vi "LabVIEW Gaussian Signal Monitor with UDP Alert System.vi"() -> ()   [LabVIEW 2024]
uses:
  Pro. Cases.ctl
  Con. Cases.ctl
  <vilib>/Utility/file.llb/Write Delimited Spreadsheet (DBL).vi
panel:
  out "error out":errorcluster
  in  "S. Freq. (Hz)":dbl=10.0 min=10.0 max=200.0
  out "Triggered Data":dbl[](graph)
  out "Real Time":dbl(graph)
  in  "L (V)":dbl=0.0001 min=0.0001 max=0.9999
  in  "W (s)":dbl min=1.0001
  in  "K (s)":dbl min=0.0001
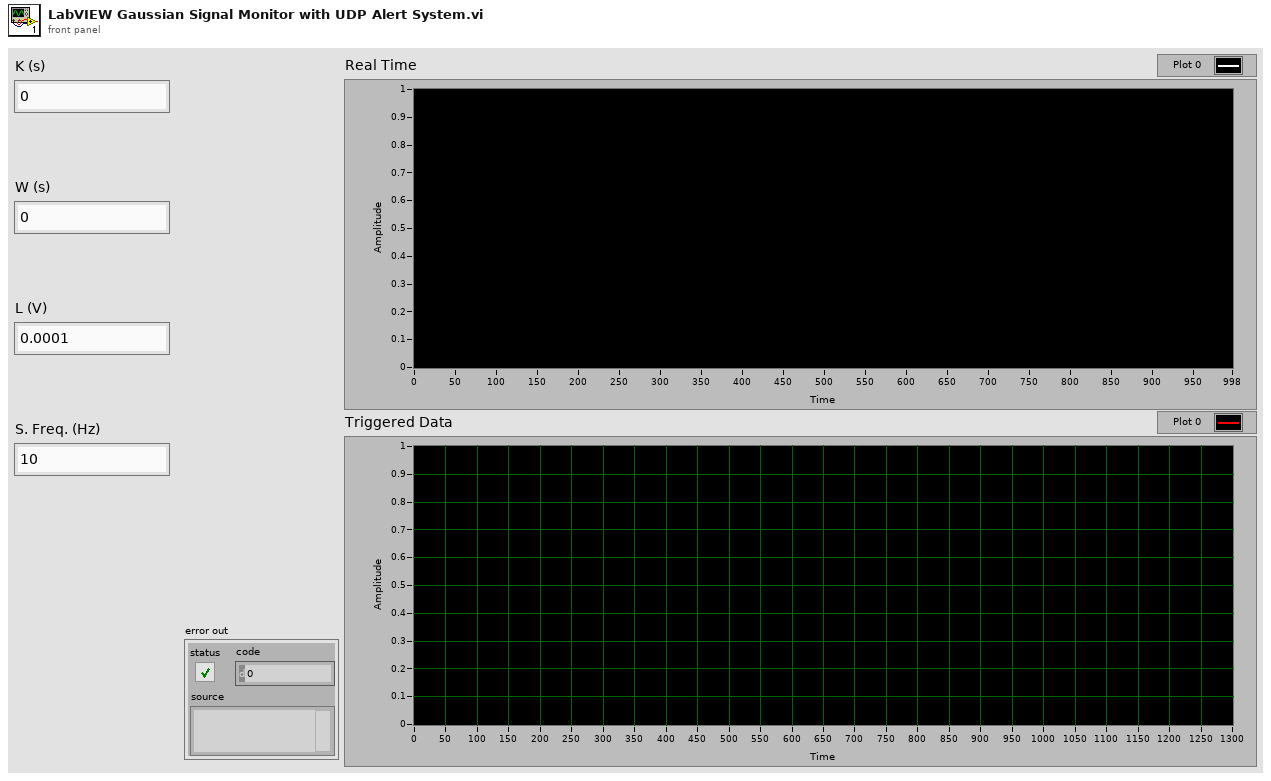
[diagram p1: front panel]
types:
  T1 = typedef "Con. Cases.ctl" = enum16{"Transmission", "Stop"}
  T2 = enum16{"open", "replace", "create", "open or create", "replace or create", "replace or create with confirmation"}
  T3 = typedef "Pro. Cases.ctl" = enum16{"Poll", "Acq.", "Save", "Stop"}
  T4 = cluster{"Pro. Cases":T3, "W (s)":dbl, "L (V)":dbl, "K (s)":dbl, "S. Freq. (Hz)":dbl, "i":dbl, "x (t)":dbl, "Trg.":bool, "counter":i32, "Trg. F.":dbl[], "File":refnum<file>}
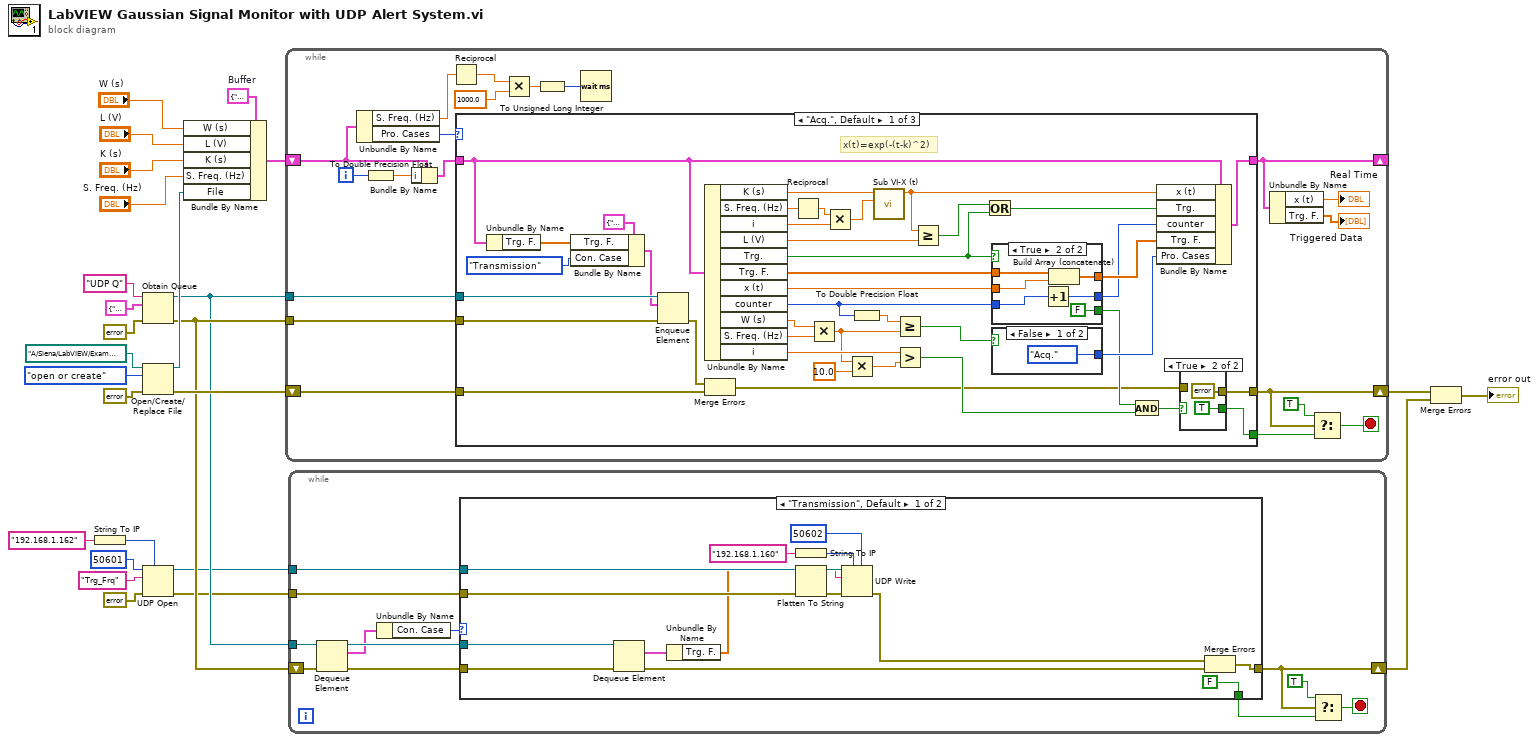
[diagram p0: block diagram]
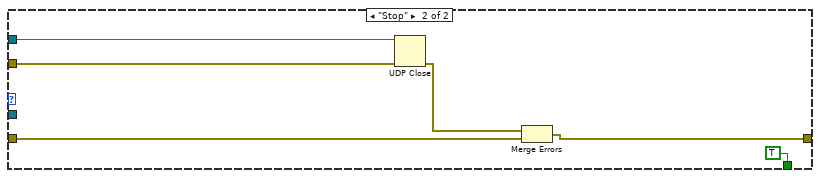
[diagram p2: hidden frame]
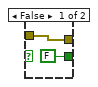
[diagram p3: hidden frame]
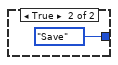
[diagram p4: hidden frame]
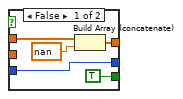
[diagram p5: hidden frame]
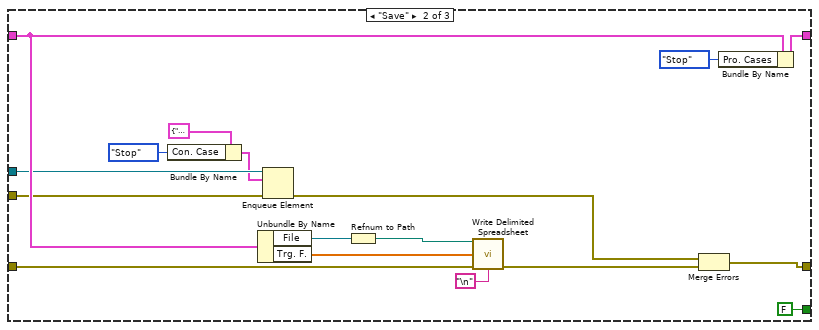
[diagram p6: hidden frame]
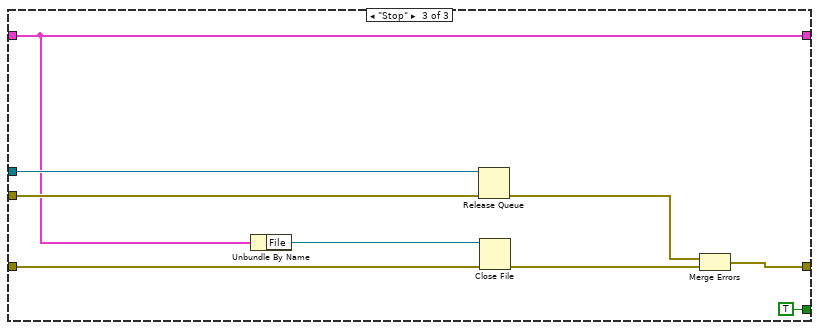
[diagram p7: hidden frame]
diagram:
  w26 = T4 {"Pro. Cases"=enum."Acq.", "W (s)"=0.0, "L (V)"=0.0, "K (s)"=0.0, "S. Freq. (Hz)"=0.0, "i"=0.0, "x (t)"=0.0, "Trg."=FALSE, "counter"=0, "Trg. F."=[], "File"=refnum}  # Buffer
  n1 = String To IP(1:"192.168.1.162" ("name")) -> (0:w2:u32)
  n2 = Obtain Queue(name (unnamed)="UDP Q", element data type=cluster{"Con. Case":T1, "Trg. F.":dbl[]} {"Con. Case"=enum."Transmission", "Trg. F."=[]}, error in (no error)=errorcluster {"status"=FALSE, "code"=0, "source"=""} ("error in")) -> (queue out=w11:refnum<queue>, error out=w12:errorcluster)  [unwired: 2 in, 1 out]
  n3 = Open/Create/Replace File(file path (use dialog)=path "A:/Siena/LabVIEW/Exam Perp/Triggered Data/Trg data.csv", error in=errorcluster {"status"=FALSE, "code"=0, "source"=""}, operation (0:open)=T2."open or create") -> (refnum out=w16:refnum<file>, error out=w17:errorcluster)  [unwired: 3 in, 1 out]
  n4 = UDP Open(7:w2, 8:errorcluster {"status"=FALSE, "code"=0, "source"=""} ("error in"), 10:"Trg_Frq" ("service name"), 11:u16 50601 ("port")) -> (port=w7:refnum<k16>, 0:w6:errorcluster)  [unwired: 1 in, 1 out]
  n5 = Bundle By Name(cluster=w26, "W (s)"="W (s)", "L (V)"="L (V)", "K (s)"="K (s)", "S. Freq. (Hz)"="S. Freq. (Hz)", "File"=w16) -> (w25:T4)
  n6 = while {
    shift-right: [w36] -> _
    shift-left: w25 -> [w40]
    shift-right: [w32] -> w15
    shift-left: w17 -> [w33]
    tunnel: w11 -> [w28]
    tunnel: w12 -> [w27]
    i -> [w46]
    stop <- w29 stop-if-true
    n7 = Unbundle By Name(w40) -> ("S. Freq. (Hz)"=w41:dbl, "Pro. Cases"=w38:T3)
    n8 = To Double Precision Float(number=w46) -> (double precision float=w37:dbl)
    n9 = Bundle By Name(cluster=w40, "i"=w37) -> (w39:T4)
    n10 = Reciprocal(x=w41) -> (1/x=w42:dbl)
    n11 = case shown="\"Acq.\", Default" w38 {
      tunnel: w39 -> [w49 w120 w121]
      tunnel: [w80 w119 w121] -> w36
      tunnel: w33 -> [w54 w116 w129]
      tunnel: [w63 w104 w122] -> w32
      tunnel: [w62 FALSE TRUE] -> w30
      tunnel: w28 -> [w56 w111 w126]
      tunnel: w27 -> [w55 w110 w125]
      frame "Acq.", Default {
        # "x(t)=exp(-(t-k)^2)"
        n12 = Unbundle By Name(w49) -> ("Trg. F."=w48:dbl[])
        n13 = Bundle By Name(cluster=cluster{"Con. Case":T1, "Trg. F.":dbl[]} {"Con. Case"=enum."Transmission", "Trg. F."=[]}, "Trg. F."=w48, "Con. Case"=Con._Cases."Transmission") -> (w50:cluster{"Con. Case":T1, "Trg. F.":dbl[]})
        n14 = Enqueue Element(queue=w56, element=w50, error in (no error)=w55) -> (error out=w52:errorcluster)  [unwired: 1 in, 2 out]
        n15 = Unbundle By Name(w49) -> ("K (s)"=w85:dbl, "S. Freq. (Hz)"=w84:dbl, "i"=w81:dbl, "L (V)"=w79:dbl, "Trg."=w76:bool, "Trg. F."=w73:dbl[], "x (t)"=w72:dbl, "counter"=w69:i32, "W (s)"=w71:dbl, "S. Freq. (Hz)"=w70:dbl, "i"=w61:dbl)
        n16 = Merge Errors(w52, w54) -> (w53:errorcluster)
        n17 = Reciprocal(x=w84) -> (1/x=w83:dbl)
        n18 = Multiply(x=w71, y=w70) -> (x*y=w57:dbl)
        n19 = Multiply(x=w83, y=w81) -> (x*y=w82:dbl)
        n20 = Multiply(x=w57, y=10.0) -> (x*y=w64:dbl)
        n21 = To Double Precision Float(number=w69) -> (double precision float=w65:dbl)
        n22 = call "Sub VI-X (t).vi"("t"=w82, "K"=w85) -> ("x (t)"=w74:dbl)  [unwired: 8 in, 1 out]
        n23 = Greater Or Equal?(x=w65, y=w57) -> (x >= y?=w68:bool)
        n24 = Greater?(x=w61, y=w64) -> (0:w58:bool)
        n25 = Greater Or Equal?(x=w74, y=w79) -> (x >= y?=w78:bool)
        n26 = Or(x=w78, y=w76) -> (x .or. y?=w77:bool)
        n27 = case shown="True" w76 {
          tunnel: w69 -> [w97 w103]
          tunnel: [w97 w102] -> w75
          tunnel: w73 -> [w95 w101]
          tunnel: [w96 w100] -> w86
          tunnel: w72 -> [_ w99]
          tunnel: [TRUE FALSE] -> w59
          frame False {
            n28 = Build Array (concatenate)(w95, nan) -> (w96:dbl[])
          }
          frame True {
            n29 = Increment(x=w103) -> (x+1=w102:i32)
            n30 = Build Array (concatenate)(w101, w99) -> (w100:dbl[])
          }
        }
        n31 = case shown="False" w68 {
          tunnel: [Pro._Cases."Acq." ("Cases") Pro._Cases."Save" ("Cases")] -> w67
          frame False {
          }
          frame True {
          }
        }
        n32 = And(x=w59, y=w58) -> (x .and. y?=w60:bool)
        n33 = Bundle By Name(cluster=w49, "x (t)"=w74, "Trg."=w77, "counter"=w75, "Trg. F."=w86, "Pro. Cases"=w67) -> (w80:T4)
        n34 = case shown="True" w60 {
          tunnel: w53 -> [w88 _]
          tunnel: [w88 errorcluster {"status"=TRUE, "code"=5050, "source"="Waiting for trigger timeout error"} ("error out")] -> w63
          tunnel: [FALSE TRUE] -> w62
          frame False {
          }
          frame True {
          }
        }
      }
      frame "Save" {
        n35 = Bundle By Name(cluster=cluster{"Con. Case":T1, "Trg. F.":dbl[]} {"Con. Case"=enum."Transmission", "Trg. F."=[]} ("element"), "Con. Case"=Con._Cases."Stop") -> (w108:cluster{"Con. Case":T1, "Trg. F.":dbl[]})
        n36 = Unbundle By Name(w120) -> ("File"=w115:refnum<file>, "Trg. F."=w113:dbl[])
        n37 = Enqueue Element(queue=w111, element=w108, error in (no error)=w110) -> (error out=w105:errorcluster)  [unwired: 1 in, 2 out]
        n38 = Refnum to Path(1:w115) -> (0:w114:path)
        n39 = call-poly <vilib>:"Write Delimited Spreadsheet.vi"("file path (dialog if empty)"=w114, "1D data"=w113, "error in (no error)"=w116, "delimiter (\\t)"="\n") -> ("error out"=w106:errorcluster)  [unwired: 10 in, 1 out]
        n40 = Merge Errors(w105, w106) -> (w104:errorcluster)
        n41 = Bundle By Name(cluster=w120, "Pro. Cases"=Pro._Cases."Stop" ("Cases")) -> (w119:T4)
      }
      frame "Stop" {
        n42 = Unbundle By Name(w121) -> ("File"=w128:refnum<file>)
        n43 = Release Queue(queue=w126, error in (no error)=w125) -> (error out=w124:errorcluster)  [unwired: 1 in, 2 out]
        n44 = Close File(refnum=w128, error in=w129) -> (error out=w123:errorcluster)  [unwired: 1 out]
        n45 = Merge Errors(w124, w123) -> (w122:errorcluster)
      }
    }
    n46 = Multiply(x=w42, y=1000.0) -> (x*y=w45:dbl)
    n47 = To Unsigned Long Integer(number=w45) -> (unsigned 32bit integer=w44:u32)
    n48 = Wait (ms)(milliseconds to wait=w44) -> ()  [unwired: 1 out]
    n49 = Unbundle By Name(w36) -> ("x (t)"=→"Real Time":dbl, "Trg. F."=→"Triggered Data":dbl[])
    n50 = Select(t=TRUE, s=w32, f=w30) -> (s? t:f=w29:bool)
  }
  n51 = while {
    tunnel: w11 -> [w140]
    tunnel: w7 -> [w131]
    tunnel: w6 -> [w130]
    shift-right: [w135] -> w8
    shift-left: w12 -> [w141]
    stop <- w134 stop-if-true
    n52 = Dequeue Element(queue=w140, error in (no error)=w141) -> (queue out=w139:refnum<queue>, element=w137:cluster{"Con. Case":T1, "Trg. F.":dbl[]}, error out=w138:errorcluster)  [unwired: 1 in, 1 out]
    n53 = Unbundle By Name(w137) -> ("Con. Case"=w136:T1)
    n54 = case shown="\"Transmission\", Default" w136 {
      tunnel: w139 -> [w150 _]
      tunnel: w138 -> [w156 w162]
      tunnel: [w153 w158] -> w135
      tunnel: [FALSE TRUE] -> w132
      tunnel: w131 -> [w154 w160]
      tunnel: w130 -> [w147 w159]
      frame "Transmission", Default {
        n55 = Dequeue Element(queue=w150, error in (no error)=w156) -> (element=w149:cluster{"Con. Case":T1, "Trg. F.":dbl[]}, error out=w151:errorcluster)  [unwired: 1 in, 2 out]
        n56 = Unbundle By Name(w149) -> ("Trg. F."=w142:dbl[])
        n57 = String To IP(1:"192.168.1.160" ("name")) -> (0:w144:u32)
        n58 = Flatten To String(anything=w142, error in (no error)=w147) -> (data string=w148:string, error out=w146:errorcluster)  [unwired: 2 in, 1 out]
        n59 = UDP Write(address=w144, port or service name=u16 50602, connection ID=w154, data in=w148, 8:w146) -> (error out=w152:errorcluster)  [unwired: 1 in, 1 out]
        n60 = Merge Errors(w152, w151) -> (w153:errorcluster)
      }
      frame "Stop" {
        n61 = UDP Close(connection ID=w160, 8:w159) -> (error out=w157:errorcluster)  [unwired: 1 out]
        n62 = Merge Errors(w157, w162) -> (w158:errorcluster)
      }
    }
    n63 = Select(t=TRUE, s=w135, f=w132) -> (s? t:f=w134:bool)
  }
  n64 = Merge Errors(w15, w8) -> (→"error out":errorcluster)
